vi "Exemple_Model_Selection_GroupShuffleSplit.vi"() -> ()   [LabVIEW 2020]
panel:
  out "Split":T1(array[cluster])
  out "error out":errorcluster caption="sortie d'erreur"
  in  "GroupShuffleSplit":T2={"n_splits"=2, "test_size"="0.2", "train_size"="0.7", "random_state"=42} {"random_state" min=-1}
  in  "error in (no error)":errorcluster caption="entrée d'erreur (pas d'erreur)"
  in  "Groups":string[][](array[string])=[["1"], ["1"], ["2"], ["2"], ["2"], ["3"], ["3"], ["3"]]
  in  "y":string[][](array[string])=[["1"], ["1"], ["1"], ["1"], ["1"], ["1"], ["1"], ["1"]]
  in  "X":string[][](array[string])=[["1", "1"], ["1", "1"], ["1", "1"], ["1", "1"], ["1", "1"], ["1", "1"], ["1", "1"], ["1", "1"]]
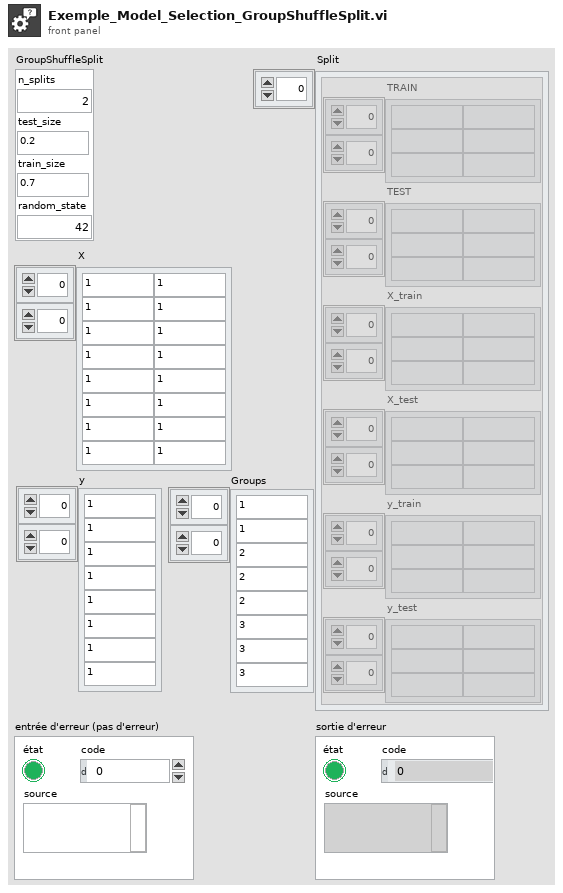
[diagram p1: front panel]
types:
  T1 = cluster{"TRAIN":string[][], "TEST":string[][], "X_train":string[][], "X_test":string[][], "y_train":string[][], "y_test":string[][]}[]
  T2 = cluster{"n_splits":i32, "test_size":string, "train_size":string, "random_state":i32}
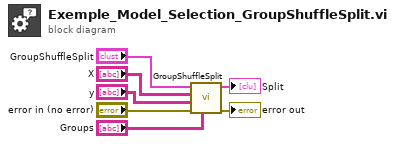
[diagram p0: block diagram]
diagram:
  n1 = call "GroupShuffleSplit.vi"("Groups"="Groups", "error in (no error)"="error in (no error)", "y"="y", "X"="X", "GroupShuffleSplit"="GroupShuffleSplit") -> ("error out"=→"error out":errorcluster, "Split"=→"Split":T1)  [unwired: 5 in]
